vi "Dispatch Message.vi"(8 "error in (no error)":errorcluster, 10 "TSnax:UIMessage":refnum<class "UIMessage.lvclass">, 11 "Engine in":refnum<class "Engine.lvclass">) -> (0 "error out":errorcluster, 3 "Engine out":refnum<class "Engine.lvclass">)   [LabVIEW 2020, in "TSnax.lvlib" / "Engine.lvclass"]
uses:
  Engine.lvclass
  UIMessage/UIMessage.lvclass
  Engine.lvclass/Engine.ctl
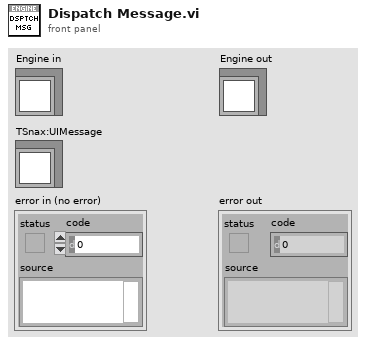
[diagram p1: front panel]
types:
  T1 = typedef "TSnax.lvlib/UIMsg.ctl" = enum16{"Unknown", "BreakOnUserRequest", "BreakOnBreakpoint", "BreakOnRunTimeError", "Trace", "TerminatingExecution", "AbortingExecution", "KillingExecutionThreads", "EndExecution", "ShutDownComplete", "StartExecution", "ProgressPercent", "ProgressText", "StartInteractiveExecution", "EndInteractiveExecution", "TerminatingInteractiveExecution", "TerminationCancelled", "ResumeFromBreak", "StartFileExecution", "EndFileExecution", "ShutDownCancelled", "LocalizationSettingChanged", "OpenWindows", "TileWindows", "CascadeWindows", "ReportChanged", "CloseWindows", "RefreshWindows", "ClientFileChanged", "DisplayReport", "ModelState_Initializing", "ModelState_Waiting", "ModelState_Identified", "ModelState_BeginTesting", "ModelState_TestingComplete", "ModelState_PostProcessingComplete", "ModelState_EnabledStateSet", "ReportLocationChanged", "GotoLocation", "PushUndoItem", "OutputMessages", "TypePaletteFileListChanged", "NonTerminatingThreadsArePreventingTermination", "ModelState_PostProcessing", "ReportCollectionChanged", "RuntimeError"}
  T2 = typedef "TSnax.lvlib/Engine.lvclass/UIMessage Callbacks.ctl" = cluster{"Callbacks":T3[], "ID Map":map{T1, i32[]}}
  T3 = typedef "TSnax.lvlib/Engine.lvclass/UIMessage Callback.ctl" = cluster{"VI":T4, "Owner":refnum<class>, "User Data":variant, "IDs":T1[]}
  T4 = typedef "TSnax.lvlib/Engine.lvclass/UIMsg Callback VI.ctl" = refnum<vi>
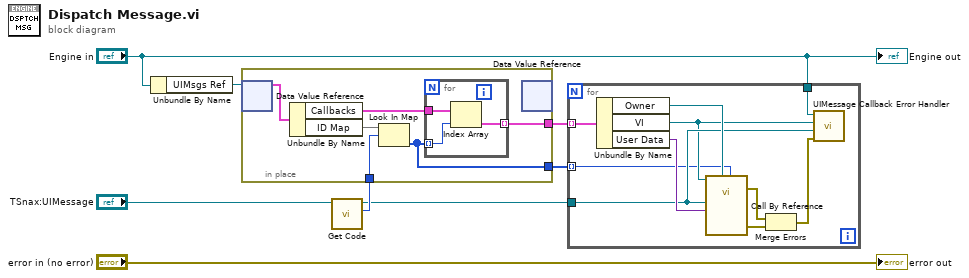
[diagram p0: block diagram]
diagram:
  n1 = Unbundle By Name("Engine in") -> ("UIMsgs Ref"=w7:refnum<data-value>)
  n2 = call "Get Code.vi"("UIMessage in"="TSnax:UIMessage") -> ("Code"=w5:T1, "UIMessage out"=w3:refnum<class "UIMessage.lvclass">)  [unwired: 8 in, 1 out]
  n3 = in-place {
    in-place-border: [w11] -> w4
    in-place-border: w5 -> [w10]
    in-place-border: [w9] -> w1
    n4 = in-place-dvr #1(w7) -> (w14:T2)  [unwired: 1 out]
    n5 = Unbundle By Name(w14) -> ("Callbacks"=w12:T3[], "ID Map"=w13:map{T1, i32[]})
    n6 = Look In Map(map=w13, key=w10) -> (value=w9:i32[])  [unwired: 1 in, 1 out]
    n7 = for {
      tunnel: w9 -> [w16] mode=indexing
      tunnel: w12 -> [w17]
      tunnel: [w15] -> w11 mode=indexing
      n8 = Index Array(array=w17, index=w16) -> (element=w15:T3)
    }
    n9 = in-place-dvr #1() -> ()  [unwired: 1 in, 2 out]
  }
  n10 = for {
    tunnel: w4 -> [w27] mode=indexing
    tunnel: w3 -> [w21]
    tunnel: "Engine in" -> [w19]
    tunnel: w1 -> [w18] mode=indexing
    n11 = Unbundle By Name(w27) -> ("Owner"=w25:refnum<class>, "VI"=w20:T4, "User Data"=w26:variant)
    n12 = call-by-ref "?"(reference=w20, "Callback ID"=w18, "Owner"=w25, "User Data"=w26, "UIMessage"=w21) -> (error out=w23:errorcluster, 0:"error out"=w24:errorcluster)  [unwired: 8 in, 1 out]
    n13 = Merge Errors(w23, w24) -> (w22:errorcluster)
    n14 = call "UIMessage Callback Error Handler.vi"("error in (no error)"=w22, "TSnax:UIMessage"=w21, "VI"=w20, "TSnax:Engine"=w19) -> ()  [unwired: 8 in]
  }
  "error out" <- "error in (no error)"
  "Engine out" <- "Engine in"
